vi "ConfigPhases.vi"(8 "error in (no error)":errorcluster, 11 "NhRegenGridSim in":refnum<class "NHRGridSim.lvclass">) -> (0 "error out":errorcluster, 3 "NhRegenGridSim out":refnum<class "NHRGridSim.lvclass">)   [LabVIEW 2018, in "AcPwrPlugins.lvlib" / "NHRGridSim.lvclass"]
doc: "This VI sets the selected logical instrument to apply changes at the set phase angle when operating with synchronization enabled using Configure Synchronization.vi.\n\nThis command ONLY applies to an instrument in AC mode."
uses:
  NHRGridSim.lvclass
  <instrlib>/NH Research 9400 Series/NH Research 9400 Series.lvlib
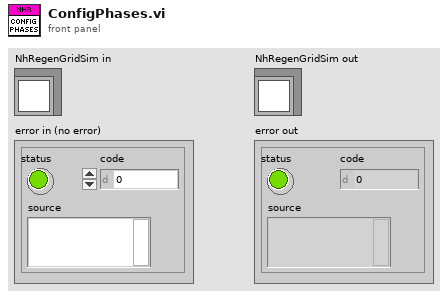
[diagram p1: front panel]
types:
  T1 = typedef "AcPwrPlugins.lvlib/NHRGridSim.lvclass/Device(s)Settings.ctl" = cluster{"MeasName":string, "Modules":T2}
  T2 = typedef "AcPwrPlugins.lvlib/NHRGridSim.lvclass/Modules.ctl" = cluster{"Measurement":cluster{"ApertureLength (s)":dbl, "NumberOfSamples":u32}, "Ranges":cluster{"Irange (A)":dbl, "Vrange (V)":dbl}, "Mode":u8, "Handle":string, "FreqOut (Hz)":dbl, "Connected":bool, "btnIdQuery":bool, "btnReset":bool, "Initialize Timeout ( ms)":u32, "Phase (0: All)":i32, "WatchDog":cluster{"Enable WatchDog":bool, "Robust WatchDog":bool, "Watchdog Interval (s)":dbl}, "Safety Limits":cluster{"Min Voltage (V)":dbl, "Min Voltage Time (s)":dbl, "Max Voltage (V)":dbl, "MaxVoltage Time (s)":dbl, "Max Source Amps (A)":dbl, "Max Source Amps Time (s)":dbl, "Max Sink Amps (A)":dbl, "Max Sink Amps Time (s)":dbl, "Max Source Power (W)":dbl, "Max Source Power Time (s)":dbl, "Max Sink Power (W)":dbl, "Max Sink Power Time (s)":dbl, "Peak Voltage (V)":dbl, "Peak Voltage Enable":bool, "Peak Amps (A)":dbl, "Peak Amps Enable":bool}, "Phases":cluster{"Pout (W)":dbl, "Iout (A)":dbl, "PhaseAngle":dbl, "Vout (V)":dbl, "Phase Name":string}[], "Regulation Gain":dbl, "ChangeOntheFly":bool, "Synchronize Output \nto Phase":bool, "Slew Rate":cluster{"Voltage Slew (Volts/s)":dbl, "Phase Angle (Degrees/s)":dbl}}[]
  T3 = enum8{"One 3-Phase AC", "One AC", "One DC", "Three AC", "Three DC", "One 2-Phase AC and One AC", "One 2-Phase AC and One DC", "Two AC", "One AC and One DC", "Two AC and One DC", "One AC and Two DC", "One DC and One AC", "Two DC"}
  T4 = cluster{"Pout (W)":dbl, "Iout (A)":dbl, "PhaseAngle":dbl, "Vout (V)":dbl, "Phase Name":string}[]
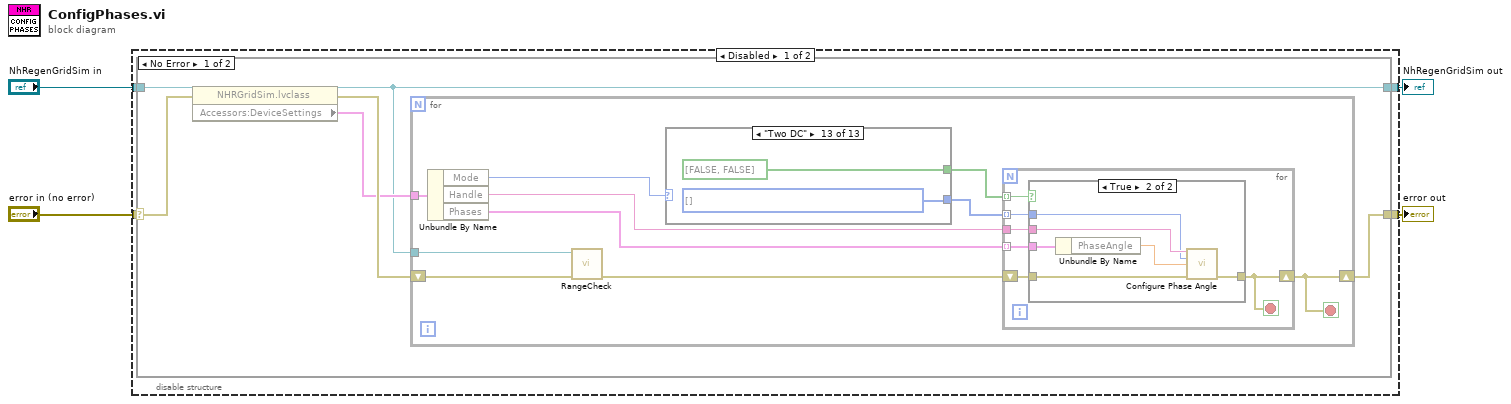
[diagram p0: block diagram]
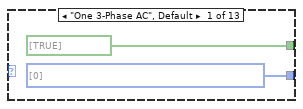
[diagram p2: hidden frame]
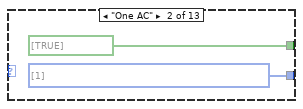
[diagram p3: hidden frame]
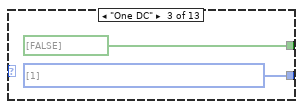
[diagram p4: hidden frame]
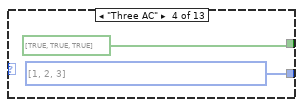
[diagram p5: hidden frame]
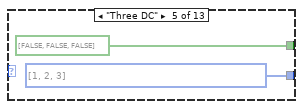
[diagram p6: hidden frame]
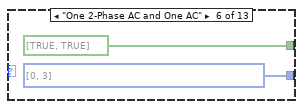
[diagram p7: hidden frame]
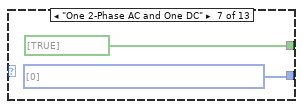
[diagram p8: hidden frame]
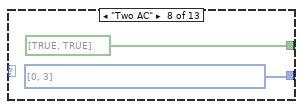
[diagram p9: hidden frame]
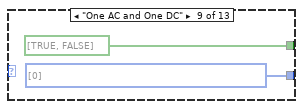
[diagram p10: hidden frame]
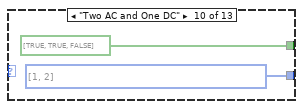
[diagram p11: hidden frame]
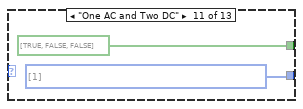
[diagram p12: hidden frame]
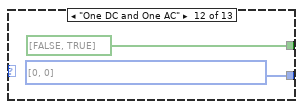
[diagram p13: hidden frame]
diagram:
  n1 = disable-structure shown="Disabled" {
    disable-tunnel: [w8 w66] -> w4
    disable-tunnel: [w7 w67] -> w3
    disable-tunnel: "error in (no error)" -> [w6 w66]
    disable-tunnel: "NhRegenGridSim in" -> [w5 w67]
    frame Disabled {
      n2 = case shown="No Error" w6 {
        selector: w6 -> [w13 w64]
        tunnel: [w11 w64] -> w8
        tunnel: [w9 w65] -> w7
        tunnel: w5 -> [w14 w65]
        frame No Error {
          n3 = property class="NHRGridSim.lvclass"(reference=w14, error in=w13) -> (reference out=w9:refnum<class "NHRGridSim.lvclass">, error out=w12:errorcluster, "Accessors:DeviceSettings"=w10:T1)
          n4 = for {
            shift-right: [w18] -> w11
            shift-left: w12 -> [w21]
            tunnel: w10 -> [w23]
            tunnel: w9 -> [w19]
            stop <- w18 stop-if-true
            n5 = Unbundle By Name(w23) -> ("Mode"=w17:T3, "Handle"=w22:string, "Phases"=w24:T4)
            n6 = call-dynamic "RangeCheck.vi"("NhRegenGridSim in"=w19, "error in (no error)"=w21) -> ("error out"=w20:errorcluster)  [unwired: 7 in, 1 out]
            n7 = case shown="\"Two DC\"" w17 {
              tunnel: [w25 w28 w29 w32 w33 w35 w37 w39 w41 w43 w46 w48 w49] -> w15
              tunnel: [bool[] [TRUE] bool[] [TRUE] bool[] [FALSE] bool[] [TRUE, TRUE, TRUE] bool[] [FALSE, FALSE, FALSE] bool[] [TRUE, TRUE] bool[] [TRUE] bool[] [TRUE, TRUE] bool[] [TRUE, FALSE] bool[] [TRUE, TRUE, FALSE] bool[] [TRUE, FALSE, FALSE] bool[] [FALSE, TRUE] bool[] [FALSE, FALSE]] -> w16
              frame "One 3-Phase AC", Default {
                w25 = i32[] [0] items=["All", "A Phase", "B Phase", "C Phase"]
              }
              frame "One AC" {
                w28 = i32[] [1] items=["All", "A Phase", "B Phase", "C Phase"]
              }
              frame "One DC" {
                w29 = i32[] [1] items=["All", "A Phase", "B Phase", "C Phase"]
              }
              frame "Three AC" {
                w32 = i32[] [1, 2, 3] items=["All", "A Phase", "B Phase", "C Phase"]
              }
              frame "Three DC" {
                w33 = i32[] [1, 2, 3] items=["All", "A Phase", "B Phase", "C Phase"]
              }
              frame "One 2-Phase AC and One AC" {
                w35 = i32[] [0, 3] items=["All", "A Phase", "B Phase", "C Phase"]
              }
              frame "One 2-Phase AC and One DC" {
                w37 = i32[] [0] items=["All", "A Phase", "B Phase", "C Phase"]
              }
              frame "Two AC" {
                w39 = i32[] [0, 3] items=["All", "A Phase", "B Phase", "C Phase"]
              }
              frame "One AC and One DC" {
                w41 = i32[] [0] items=["All", "A Phase", "B Phase", "C Phase"]
              }
              frame "Two AC and One DC" {
                w43 = i32[] [1, 2] items=["All", "A Phase", "B Phase", "C Phase"]
              }
              frame "One AC and Two DC" {
                w46 = i32[] [1] items=["All", "A Phase", "B Phase", "C Phase"]
              }
              frame "One DC and One AC" {
                w48 = i32[] [0, 0] items=["All", "A Phase", "B Phase", "C Phase"]
              }
              frame "Two DC" {
                w49 = i32[] [] items=["All", "A Phase", "B Phase", "C Phase"]
              }
            }
            n8 = for {
              tunnel: w24 -> [w55] mode=indexing
              tunnel: w22 -> [w54]
              shift-right: [w53] -> w18
              shift-left: w20 -> [w56]
              tunnel: w16 -> [w52] mode=indexing
              tunnel: w15 -> [w51] mode=indexing
              stop <- w53 stop-if-true
              n9 = case shown="True" w52 {
                tunnel: w56 -> [w57 w63]
                tunnel: w55 -> [_ w62]
                tunnel: w54 -> [_ w60]
                tunnel: [w57 w59] -> w53
                tunnel: w51 -> [_ w58]
                frame False {
                }
                frame True {
                  n10 = Unbundle By Name(w62) -> ("PhaseAngle"=w61:dbl)
                  n11 = call <instrlib>:"Configure Phase Angle.vi"("VISA resource name"=w60, "Phase (0: All)"=w58, "Phase Angle (0 Degrees)"=w61, "error in (no error)"=w63) -> ("error out"=w59:errorcluster)  [unwired: 10 in, 1 out]
                }
              }
            }
          }
        }
        frame Error {
        }
      }
    }
    frame Enabled {
    }
  }
  "error out" <- w4
  "NhRegenGridSim out" <- w3
